vi "ProcessSignals.vi"(8 "error in (no error)":errorcluster, 11 "UI Queue":refnum<queue>) -> (0 "error out":errorcluster, 2 "Array":dbl[](array[numeric]))   [LabVIEW 2018]
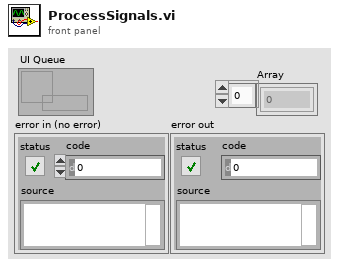
[diagram p1: front panel]
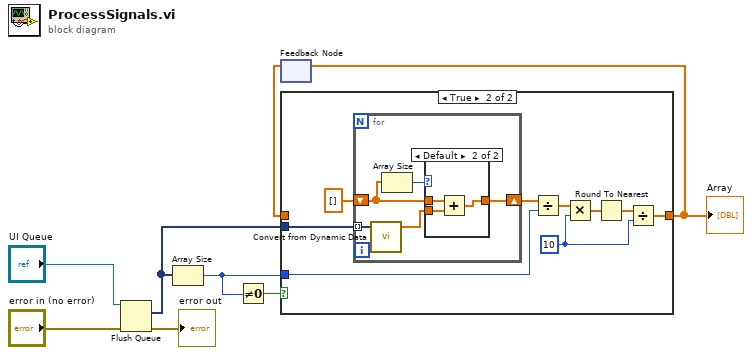
[diagram p0: block diagram]
diagram:
  n1 = Flush Queue(queue="UI Queue", error in (no error)="error in (no error)") -> (remaining elements=w4:dynamicdata[], error out=→"error out":errorcluster)  [unwired: 1 out]
  n2 = Array Size(array=w4) -> (size(s)=w3:i32)
  n3 = Not Equal To 0?(x=w3) -> (x != 0?=w5:bool)
  n4 = feedback #1() -> (w1:dbl[])  [unwired: 1 in]
  n5 = case shown="True" w5 {
    tunnel: w4 -> [_ w18]
    tunnel: w3 -> [_ w17]
    tunnel: [w9 w10] -> w2
    tunnel: w1 -> [w9 _]
    frame False {
    }
    frame True {
      w11 = 10
      n6 = for {
        tunnel: w18 -> [w23] mode=indexing
        shift-right: [w20] -> w15
        shift-left: dbl[] [] -> [w21]
        n7 = call "Convert from Dynamic Data"("Dynamic Data Type"=w23) -> ("Array"=w19:dbl[])  [unwired: 3 in]
        n8 = Array Size(array=w21) -> (size(s)=w22:i32)
        n9 = case shown="Default" w22 {
          tunnel: w21 -> [_ w25]
          tunnel: [w24 w27] -> w20
          tunnel: w19 -> [w24 w26]
          frame 0 {
          }
          frame Default {
            n10 = Add(x=w25, y=w26) -> (x+y=w27:dbl[])
          }
        }
      }
      n11 = Divide(x=w15, y=w17) -> (x/y=w12:dbl[])
      n12 = Multiply(x=w12, y=w11) -> (x*y=w14:dbl[])
      n13 = Round To Nearest(number=w14) -> (nearest integer value=w13:dbl[])
      n14 = Divide(x=w13, y=w11) -> (x/y=w10:dbl[])
    }
  }
  "Array" <- w2
  n15 = feedback-in #1(w2) -> ()
